vi "Flatten.vi"(8 "error in (no error)":errorcluster, 11 "IPacket in":refnum<class "IPacket.lvclass">) -> (0 "error out":errorcluster, 3 "Flattened Packet":string)   [LabVIEW 2020, in "MessagingInterfaces.lvlib" / "IPacket.lvclass"]
uses:
  <vilib>/gpm_packages/@cs/Network-interface/Source/MessagingInterfaces/IPacket/IPacket.lvclass
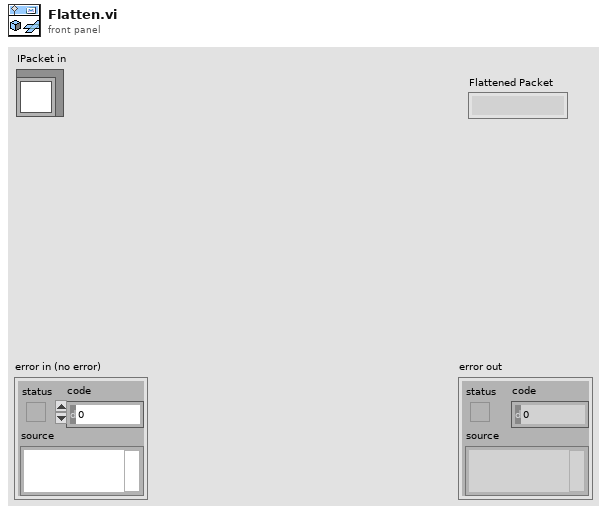
[diagram p1: front panel]
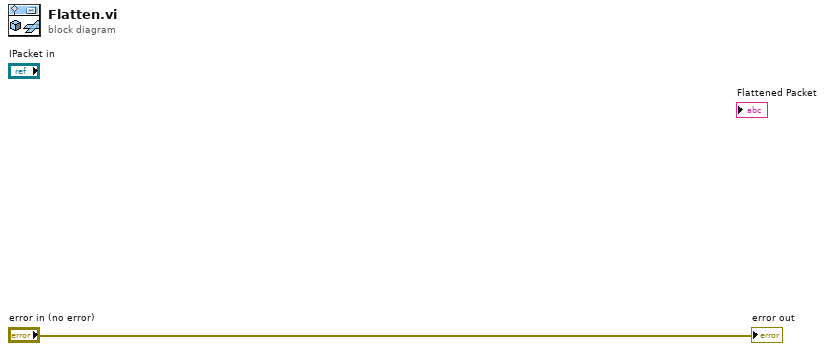
[diagram p0: block diagram]
diagram:
  "error out" <- "error in (no error)"
